vi "Project Cmd Combin.vi"(8 "error in (no error)":errorcluster, 10 "Cmd Step":T2[](array[typedef])=[enum."commamd1", enum."commamd2", enum."commamd3"], 11 "Content Input":string[](array[string])) -> (0 "error out":errorcluster, 2 "befor combine":T1, 3 "concatenated string":string)   [LabVIEW 2019]
uses:
  Ctrl/ProjectCmdStep.ctl
  Ctrl/ProjectAct Step.ctl
  Ctrl/ProjectStepSelect.ctl
  Global/Process Global.vi
panel:
  out "subarray":string[](array[string])
  in  "Cluster 2":T1
  out "element 7":string
  out "element 6":string
  out "element 5":string
  out "Array":string[](array[string])
  out "element 4":string
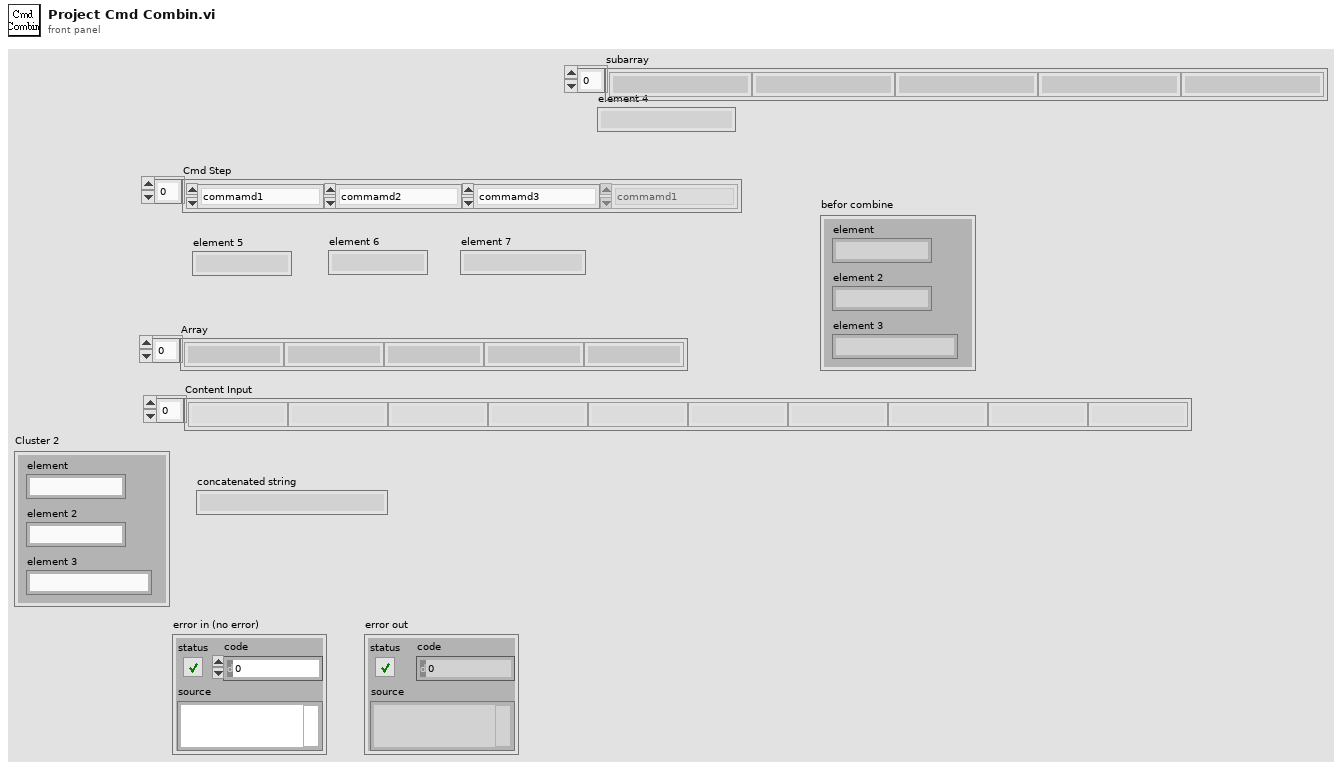
[diagram p1: front panel]
types:
  T1 = cluster{"element":string, "element 2":string, "element 3":string}
  T2 = typedef "ProjectCmdStep.ctl" = enum16{"Project Name", "commamd1", "commamd2", "commamd3", "wat time1", "return1", "return2", "return3", "wat time2", "over time", "retry"}
  T3 = typedef "ProjectAct Step.ctl" = enum16{"ProjectName", "Name", "Initial", "Reset", "Format", "Program1", "Program2", "Scan"}
  T4 = typedef "ProjectStepSelect.ctl" = enum16{"ProjectName", "Name", "Initial", "Reset", "Format", "Program1", "Program2", "Scan", "Finish", "MToolWork", "DataCheck", "DataSave", "OutputPLC", "WaitInputS1", "WaitInputOff"}
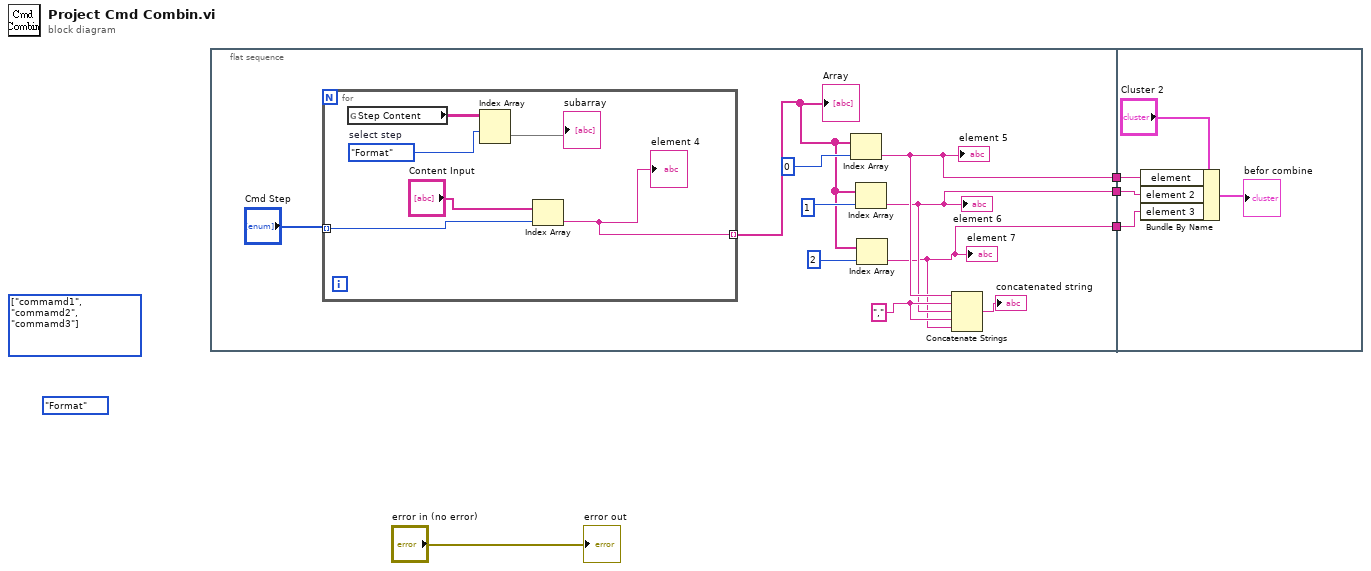
[diagram p0: block diagram]
diagram:
  (unwired) T2[] [enum."commamd1", enum."commamd2", enum."commamd3"] items=["Project Name", "commamd1", "commamd2", "commamd3", "wat time1", "return1", "return2", "return3", "wat time2", "over time", "retry"]
  (unwired) ProjectAct_Step."Format" ("select step")
  n1 = flat-sequence {
    tunnel: [w7] -> w3
    tunnel: [w6] -> w2
    tunnel: [w5] -> w1
    tunnel: w3 -> [w25]
    tunnel: w2 -> [w23]
    tunnel: w1 -> [w22]
    frame #0 {
      w9 = ","
      n2 = for {
        tunnel: "Cmd Step" -> [w20] mode=indexing
        tunnel: [w17] -> w10 mode=indexing
        w19 = ProjectStepSelect."Format"  # select step
        n3 = global read "Process Global.vi" "Step Content"() -> (w18:string[][])
        n4 = Index Array(array=w18, index (row)=w19) -> (element=→"subarray":string[])  [unwired: 1 in]
        n5 = Index Array(array="Content Input", index=w20) -> (element=w17:string)
        "element 4" <- w17
      }
      "Array" <- w10
      n6 = Index Array(array=w10, index=0) -> (element=w7:string)
      "element 5" <- w7
      n7 = Index Array(array=w10, index=1) -> (element=w6:string)
      "element 6" <- w6
      n8 = Index Array(array=w10, index=2) -> (element=w5:string)
      "element 7" <- w5
      n9 = Concatenate Strings(w7, w9, w6, w9, w5) -> (→"concatenated string":string)
    }
    frame #1 {
      n10 = Bundle By Name(cluster="Cluster 2", "element"=w25, "element 2"=w23, "element 3"=w22) -> (→"befor combine":T1)
    }
  }
  "error out" <- "error in (no error)"
